vi "rqcBob Read Channel Test Results.vi"(0 "rqcBob in":refnum<class "rqcBob.lvclass">, 9 "Timeout (ms)":u32=5000, 11 "error in (no error)":errorcluster) -> (4 "rqcBob out":refnum<class "rqcBob.lvclass">, 6 "Detections Destribution":T1, 15 "error out":errorcluster)   [LabVIEW 2018, in "rqcBob.lvclass"]
uses:
  rqcBob.lvclass
  <vilib>/Utility/error.llb/Error Cluster From Error Code.vi
  <vilib>/ErrorRing/Error Ring.xnode
  <vilib>/Analysis/NI_AALBase.lvlib
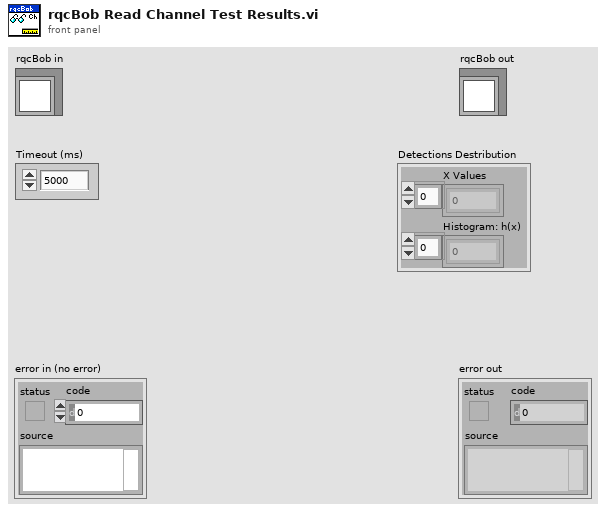
[diagram p1: front panel]
types:
  T1 = cluster{"X Values":dbl[], "Histogram: h(x)":i32[]}
  T2 = typedef "rqcBob.lvclass/rqcBob Operation Mode.ctl" = enum16{"Not Set", "Channel Test", "Key Distribution", "Modulation Level Test", "Window Test", "Delay Line Test", "Alice Modulation Level Test"}
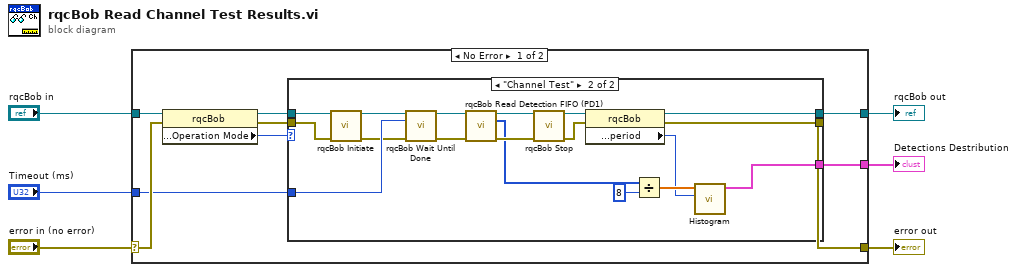
[diagram p0: block diagram]
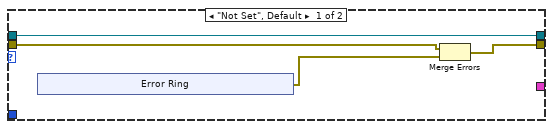
[diagram p2: hidden frame]
diagram:
  n1 = case shown="No Error" "error in (no error)" {
    selector: "error in (no error)" -> [w14 w44]
    tunnel: [w9 w44] -> w5
    tunnel: [w12 w43] -> w3
    tunnel: "rqcBob in" -> [w15 w43]
    tunnel: "Timeout (ms)" -> [w8 _]
    tunnel: [w7 _] -> w1
    frame No Error {
      n2 = property class="rqcBob"(reference=w15, error in=w14) -> (reference out=w13:refnum<class "rqcBob.lvclass">, error out=w10:errorcluster, "public:Public Properties Access:Operation Mode"=w11:T2)
      n3 = case shown="\"Channel Test\"" w11 {
        tunnel: [w19 w32] -> w12
        tunnel: w13 -> [w19 w42]
        tunnel: w10 -> [w17 w41]
        tunnel: [w18 w30] -> w9
        tunnel: w8 -> [_ w39]
        tunnel: [_ w29] -> w7
        frame "Not Set", Default {
          n4 = xnode "Error Ring"() -> ("error out"=w16:errorcluster)
          n5 = Merge Errors(w17, w16) -> (w18:errorcluster)
        }
        frame "Channel Test" {
          n6 = call-dynamic "rqcBob Initiate.vi"("rqcBob in"=w42, "error in (no error)"=w41) -> ("rqcBob out"=w40:refnum<class "rqcBob.lvclass">, "error out"=w38:errorcluster)  [unwired: 12 in]
          n7 = call-dynamic "rqcBob Wait Until Done.vi"("rqcBob in"=w40, "Timeout (ms)"=w39, "error in (no error)"=w38) -> ("rqcBob out"=w37:refnum<class "rqcBob.lvclass">, "error out"=w35:errorcluster)  [unwired: 11 in]
          n8 = call "rqcBob Read Detection FIFO (PD1).vi"("rqcBob in"=w37, "error in (no error)"=w35) -> ("rqcBob out"=w36:refnum<class "rqcBob.lvclass">, "Data"=w28:u32[], "error out"=w34:errorcluster)  [unwired: 10 in, 1 out]
          n9 = call-dynamic "rqcBob Stop.vi"("rqcBob in"=w36, "error in (no error)"=w34) -> ("rqcBob out"=w33:refnum<class "rqcBob.lvclass">, "error out"=w31:errorcluster)  [unwired: 12 in]
          n10 = property class="rqcBob"(reference=w33, error in=w31) -> (reference out=w32:refnum<class "rqcBob.lvclass">, error out=w30:errorcluster, "public:Public Properties Access:Train:period"=w25:u16)
          n11 = Divide(x=w28, y=u16 8 ("Train: Period")) -> (x/y=w27:dbl[])
          n12 = call <vilib>:"Histogram.vi"("intervals"=w25, "X"=w27) -> ("Histogram Graph"=w29:T1)  [unwired: 6 in, 3 out]
        }
      }
    }
    frame Error {
    }
  }
  "error out" <- w5
  "rqcBob out" <- w3
  "Detections Destribution" <- w1
